vi "PicoScope3000aExampleBlockAdvancedTrig.vi"() -> ()   [LabVIEW 2010]
uses:
  shared/PicoBuffers.ctl
  <vilib>/Waveform/DWDTOps.llb/DWDT Analog to Digital.vi
  shared/Buffer and Transfer Settings.ctl
  shared/Acquisition Settings.ctl
  PicoScope3000aLib/PicoScope3000aDigitalChannelSettings.ctl
  PicoScope3000aLib/PicoScope3000aAnalogChannelSettings.ctl
panel:
  in  "roundFaster":bool=TRUE
  in  "timeIntervalRequested":dbl min=0.0 format="%#6_6p"
  in  "Write to TDMS":bool
  in  "Channel B Trigger Properties":T1={"thresholdUpper"=0, "thresholdUpperHysteresis"=1024, "thresholdLower"=0, "thresholdLowerHysteresis"=1024, "Threshold Mode"=0, "Direction"=2, "Available"=FALSE} {"Direction" items=["Above / Inside", "Below / Outside", "Rising / Enter", "Falling / Exit", "Rising or Falling / Enter or Exit", "Above Lower", "Below Lower", "Rising Lower", "Falling Lower", "Positive Runt", "Negative Runt"]; "Threshold Mode" items=["Level", "Window"]}
  in  "Channel B Settings":T2={"Enabled"=FALSE, "Coupling"=1, "Range"=6, "Analogue Offset"=0.0, "Bandwidth Limit"=0} {"Bandwidth Limit" items=["Full", "20MHz"]; "Range" items=["10 mV", "20 mV", "50 mV", "100 mV", "200 mV", "500 mV", "1 V", "2 V", "5 V", "10 V", "20 V", "50 V ", "100 V"]; "Coupling" items=["AC", "DC"]}
  in  "Pulse Width Qualifier Conditions":T3 {"Condition Logic" items=["AND", "OR", "XOR"]}
  in  "Pulse Width Qualifier Settings":T4={"Direction"=2, "Lower Limit"=0, "Upper Limit"=0, "Pulse Width Type"=0} {"Pulse Width Type" items=["None", "Less Than", "Greater Than", "In Range", "Out of Range"]; "Direction" items=["Rising"=2, "Falling"=3]}
  in  "Auto Trigger (ms)":i32=1000
  in  "Trigger Conditions":T5 {"Condition Logic" items=["AND", "OR", "XOR"]}
  in  "Channel A Trigger Properties":T1={"thresholdUpper"=0, "thresholdUpperHysteresis"=1024, "thresholdLower"=0, "thresholdLowerHysteresis"=1024, "Threshold Mode"=0, "Direction"=2, "Available"=FALSE} {"Direction" items=["Above / Inside", "Below / Outside", "Rising / Enter", "Falling / Exit", "Rising or Falling / Enter or Exit", "Above Lower", "Below Lower", "Rising Lower", "Falling Lower", "Positive Runt", "Negative Runt"]; "Threshold Mode" items=["Level", "Window"]}
  in  "Digital Port  0":T6 {"Direction Channel 7" items=["Don't Care", "Low", "High", "Rising", "Falling"]; "Direction Channel 6" items=["Don't Care", "Low", "High", "Rising", "Falling"]; "Direction Channel 5" items=["Don't Care", "Low", "High", "Rising", "Falling"]; "Direction Channel 4" items=["Don't Care", "Low", "High", "Rising", "Falling"]; "Direction Channel 3" items=["Don't Care", "Low", "High", "Rising", "Falling"]; "Direction Channel 2" items=["Don't Care", "Low", "High", "Rising", "Falling"]; "Direction Channel 1" items=["Don't Care", "Low", "High", "Rising", "Falling"]; "Direction Channel 0" items=["Don't Care", "Low", "High", "Rising", "Falling"]}
  in  "Channel A Settings":T2={"Enabled"=TRUE, "Coupling"=1, "Range"=6, "Analogue Offset"=0.0, "Bandwidth Limit"=0} {"Bandwidth Limit" items=["Full", "20MHz"]; "Range" items=["10 mV", "20 mV", "50 mV", "100 mV", "200 mV", "500 mV", "1 V", "2 V", "5 V", "10 V", "20 V", "50 V ", "100 V"]; "Coupling" items=["AC", "DC"]}
  in  "Port 0 Settings":T7={"Enabled"=FALSE, "Logic Level"=9830} {"Logic Level" items=["1.5V TTL"=9830, "2.5V CMOS"=16383]}
  out "overflow":i16 format="%010b"
  in  "Apply Settings":bool
  out "USB 3.0 device on non-USB 3.0 Port":bool=TRUE
  out "USB Powered":bool=TRUE
  out "Device Info":T8={"Driver Version"="", "USB Version"="", "Hardware"="1", "Variant"="", "Batch and Serial"="", "Cal Date"="", "Kernel Version"="", "Digital HW Version"="", "Analogue HW Version"="", "MSO"=FALSE, "Number of channels"=2}
  out "error out":errorcluster
  in  "Data file":path=path "PicoScope3000aExampleBlock Data"
  in  "Buffer and Transfer Settings":T9={"startIndex"=0, "Samples"=1000000, "Down Sample Ratio"=1, "Down-Sample Mode"=0} {"Down-Sample Mode" items=["RAW none"=2147483648, "None"=0, "Aggregate"=1, "Decimate"=2, "Average"=4]; "Down Sample Ratio" step=1; "Samples" format="%_6p"}
  in  "Acquisition Settings":T10={"preTriggerSamples"=0, "postTriggerSamples"=1000000, "timebase"=0} {"postTriggerSamples" format="%_6p"; "preTriggerSamples" format="%_6p"}
  out "Properties Panel":T11 {"Max Total Capture Time Available (sec)" format="%.3p"; "Sample Frequency" format="%.6p"; "Sample Rate" format="%.3p"; "Max Samples Available" format="%_6p"; "Total Capture Time (sec)" format="%.3p"}
  out "Port 0":digitalwaveform(graph)={"t0"=timestamp(0 s since 1904-01-01), "dt"=8e-09, "Y"={"transitions"=[], "data"=[]}}
  in  "stop":bool
  out "Analog Channels":cluster{i32, sgl, "Data":dbl[]}[](graph)
  in  "Serial Number":string
  in  "Use Serial Number":bool
  in  "error in (no error)":errorcluster
  # "Bit 0 = ChA"
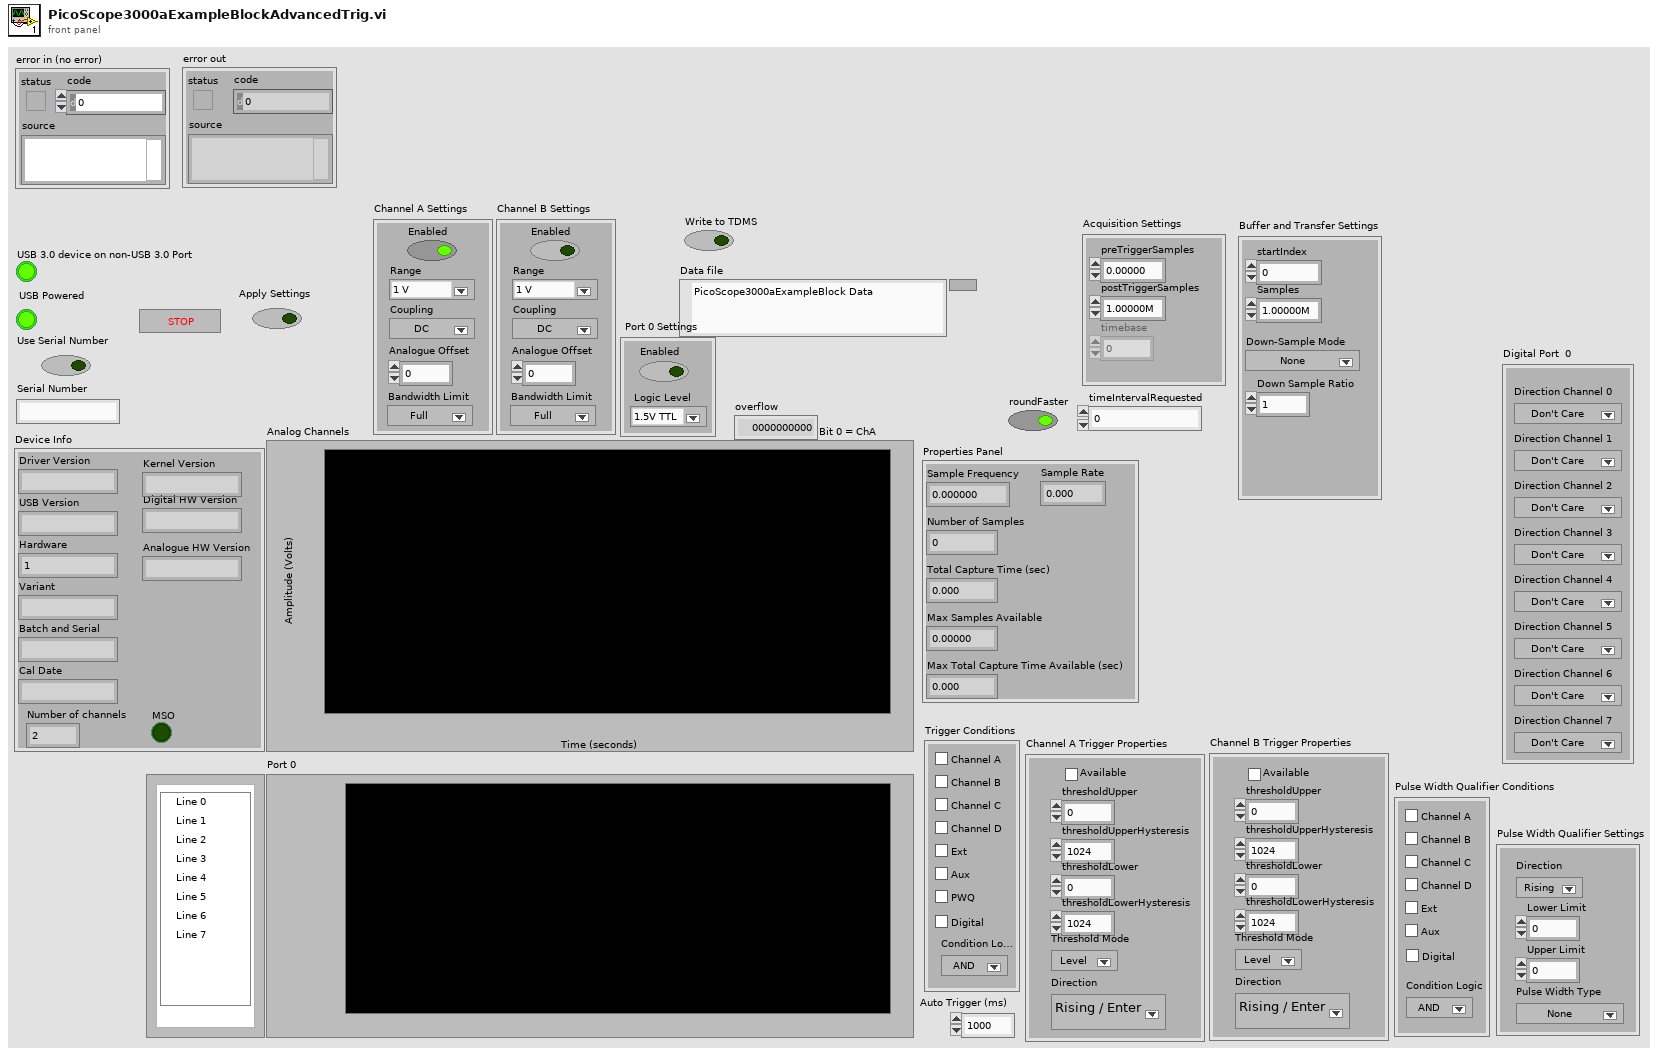
[diagram p1: front panel]
types:
  T1 = cluster{"thresholdUpper":i16, "thresholdUpperHysteresis":u16, "thresholdLower":i16, "thresholdLowerHysteresis":u16, "Threshold Mode":i32, "Direction":i32, "Available":bool}
  T2 = typedef "PicoScope3000aAnalogChannelSettings.ctl" = cluster{"Enabled":bool, "Coupling":u32, "Range":u32, "Analogue Offset":sgl, "Bandwidth Limit":u32}
  T3 = cluster{"Channel A":bool, "Channel B":bool, "Channel C":bool, "Channel D":bool, "Aux":bool, "Condition Logic":u16, "Ext":bool, "Digital":bool}
  T4 = cluster{"Direction":u32, "Lower Limit":u32, "Upper Limit":u32, "Pulse Width Type":u32}
  T5 = cluster{"Channel A":bool, "Channel B":bool, "Channel C":bool, "Channel D":bool, "Aux":bool, "PWQ":bool, "Condition Logic":u16, "Ext":bool, "Digital":bool}
  T6 = cluster{"Direction Channel 0":u16, "Direction Channel 1":u16, "Direction Channel 2":u16, "Direction Channel 3":u16, "Direction Channel 4":u16, "Direction Channel 5":u16, "Direction Channel 6":u16, "Direction Channel 7":u16}
  T7 = typedef "PicoScope3000aDigitalChannelSettings.ctl" = cluster{"Enabled":bool, "Logic Level":i16}
  T8 = cluster{"Driver Version":string, "USB Version":string, "Hardware":string, "Variant":string, "Batch and Serial":string, "Cal Date":string, "Kernel Version":string, "Digital HW Version":string, "Analogue HW Version":string, "MSO":bool, "Number of channels":i16}
  T9 = typedef "Buffer and Transfer Settings.ctl" = cluster{"startIndex":u64, "Samples":u64, "Down Sample Ratio":u64, "Down-Sample Mode":u32}
  T10 = typedef "Acquisition Settings.ctl" = cluster{"preTriggerSamples":u64, "postTriggerSamples":u64, "timebase":u32}
  T11 = cluster{"Sample Frequency":dbl, "Sample Rate":dbl, "Max Samples Available":u64, "Number of Samples":u64, "Total Capture Time (sec) ":dbl, "Max Total Capture Time Available (sec)":dbl}
  T12 = typedef "PicoBuffers.ctl" = cluster{"Max Buffer Pointers":u64[][][], "Min Buffer Pointers":u64[][][], "StreamingDataInfo":cluster{"Channel":u32, "Down-Sample Mode":u32, "PICO_DATA_TYPE":enum32{"PICO_INT8_T", "PICO_INT16_T", "PICO_INT32_T", "PICO_UINT32_T", "PICO_INT64_T", ""}, "Samples":i32, "bufferIndex":u64, "startIndex":i32, "overflow":i16}[][]}
  T13 = enum16{"open", "open or create", "create or replace", "create", "open (read-only)"}
  T14 = cluster{"Sample Frequency":sgl, "Sample Rate":sgl, "Max Samples Available":i32, "Number of Samples":u32, "Total Capture Time (sec) ":sgl, "Max Total Capture Time Available (sec)":sgl}
  T15 = cluster{"Channel A Buffer":i16[], "Channel B Buffer":i16[], "Channel C Buffer":i16[], "Channel D Buffer":i16[], "Channel E Buffer":i16[], "Channel F Buffer":i16[], "Channel G Buffer":i16[], "Channel H Buffer":i16[], "Port 0 Buffer":i16[], "Port 1 Buffer":i16[]}[]
  T16 = cluster{"Channel A Buffer":i16[], "Channel B Buffer":i16[], "Channel C Buffer":i16[], "Channel D Buffer":i16[], "Channel E Buffer":i16[], "Channel F Buffer":i16[], "Channel G Buffer":i16[], "Channel H Buffer":i16[], "Port 0 Buffer":i16[], "Port 1 Buffer":i16[]}
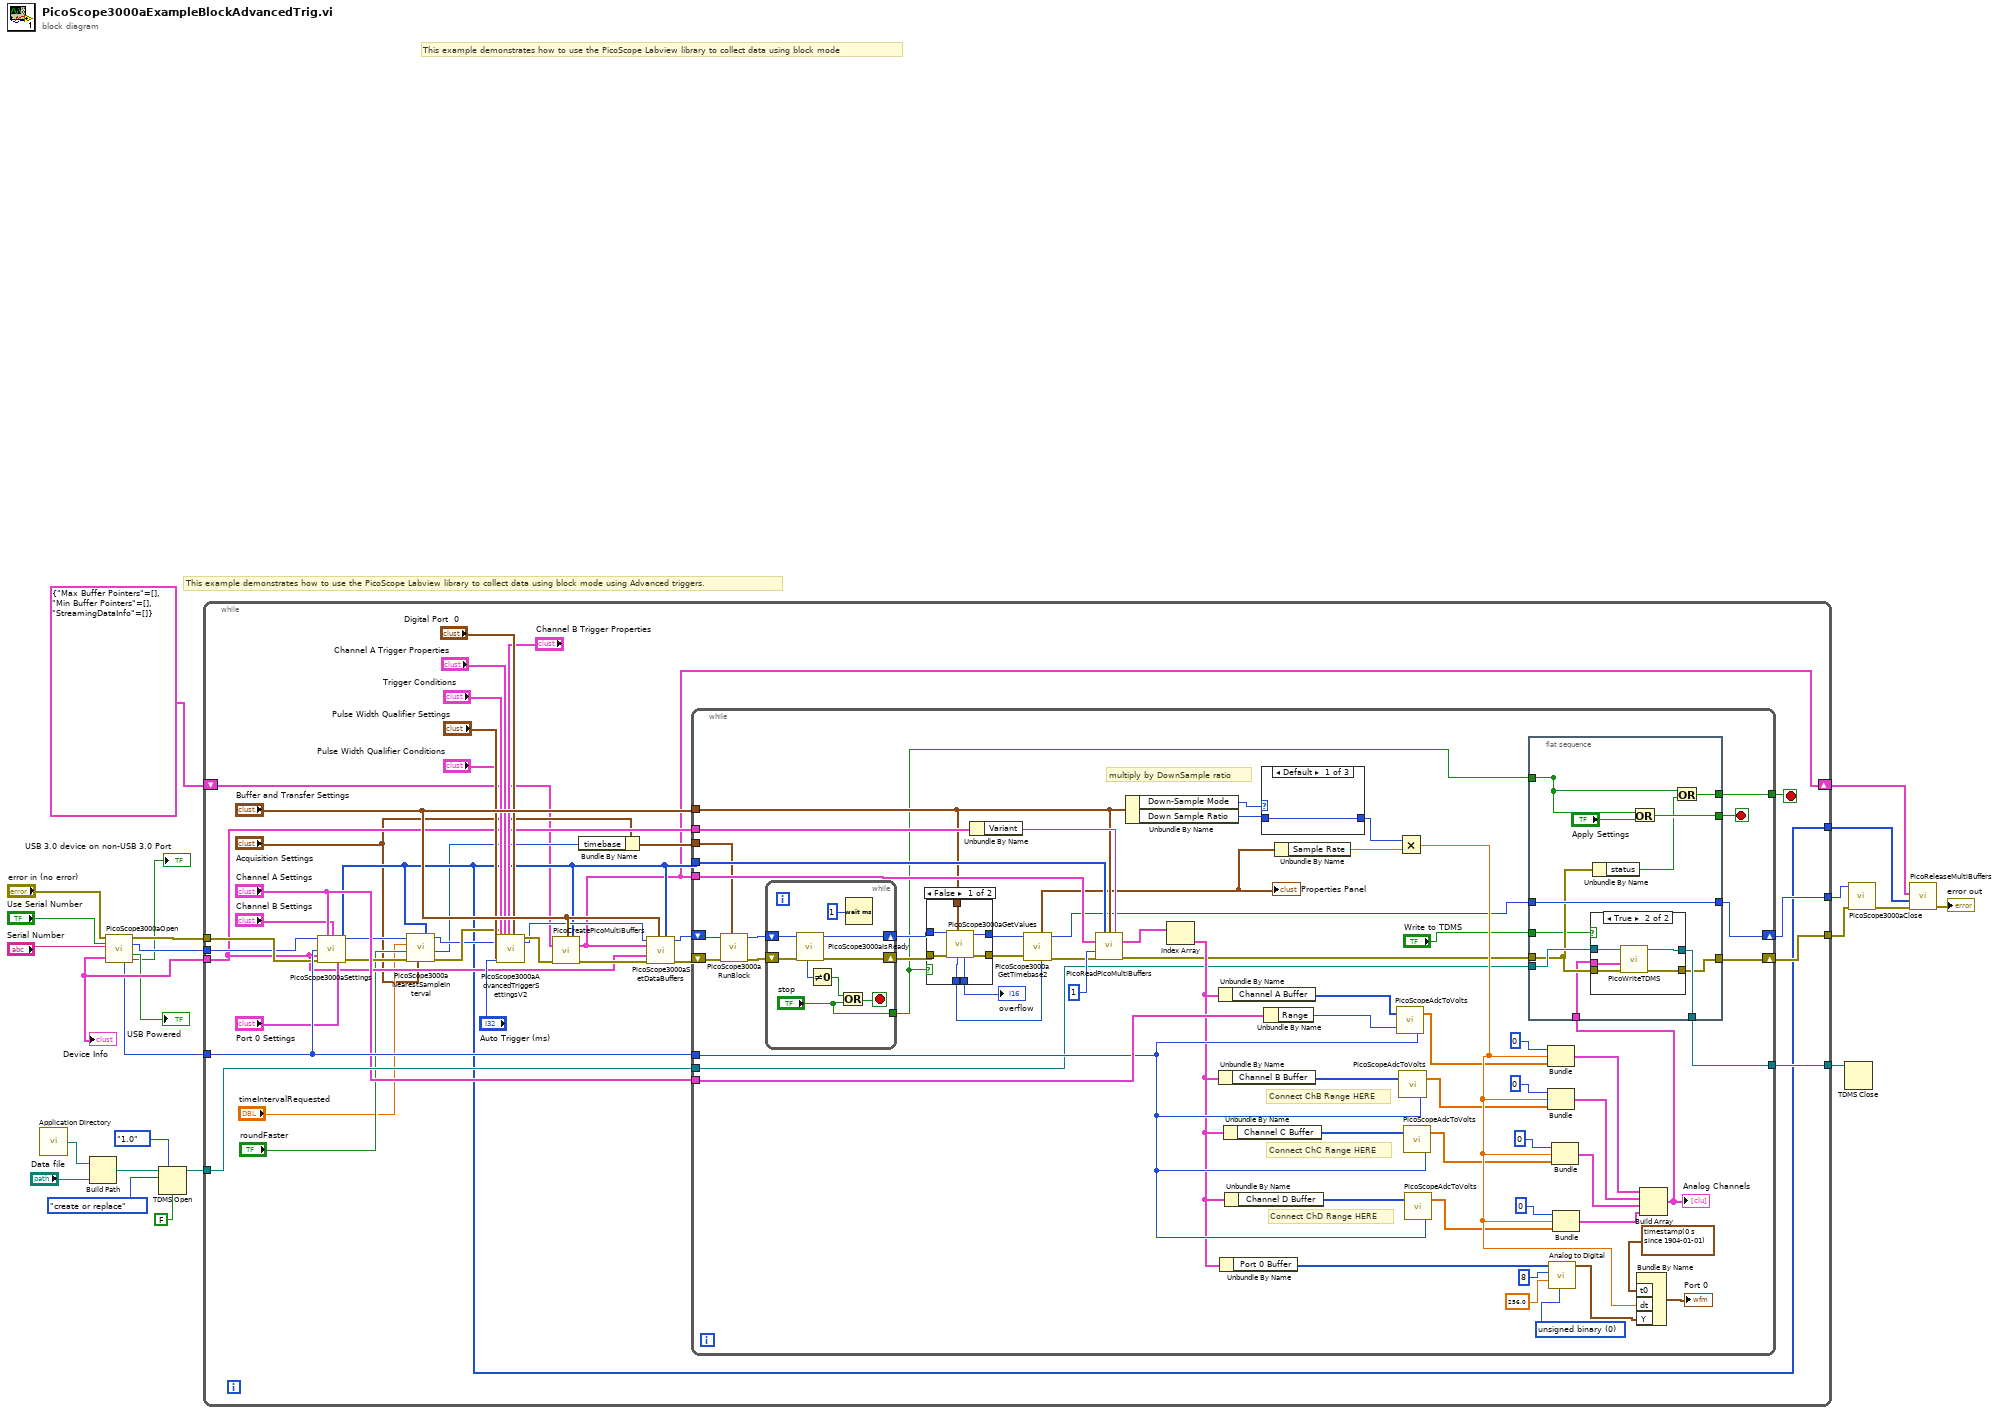
[diagram p0: block diagram]
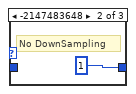
[diagram p4: hidden frame]
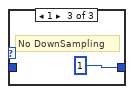
[diagram p5: hidden frame]
diagram:
  # "This example demonstrates how to use the PicoScope Labview library to collect data using block mode using Advanced triggers."
  # "This example demonstrates how to use the PicoScope Labview library to collect data using block mode"
  n1 = call <vilib>:"Application Directory.vi"() -> ("Application Directory"=w17:path)
  n2 = Build Path(base path=w17, name or relative path="Data file") -> (appended path=w18:path)
  n3 = call "PicoScope3000aOpen.vi"("error in (no error)"="error in (no error)", "Serial Number"="Serial Number", "Use Serial number"="Use Serial Number") -> ("error out"=w8:errorcluster, "handle"=w24:i16, "USB Powered"=→"USB Powered":bool, "Device Info"=w10:T8, "Max ADC value"=w6:i16, "USB 3.0 device on non-USB 3.0 Port"=→"USB 3.0 device on non-USB 3.0 Port":bool)  [unwired: 6 in, 1 out]
  "Device Info" <- w10
  n4 = TDMS Open(6:FALSE ("disable buffering? (T)"), 7:enum16{"1.0", "2.0"}."1.0" ("file format version (2.0)"), 10:T13."create or replace" ("operation (0:open)"), 11:w18) -> (3:w15:refnum<k34>)  [unwired: 2 in, 1 out]
  n5 = while {
    tunnel: w24 -> [w40]
    tunnel: w6 -> [w52]
    tunnel: [w30] -> w23
    tunnel: [w58] -> w16
    tunnel: w15 -> [w60]
    tunnel: w10 -> [w37]
    tunnel: w8 -> [w41]
    tunnel: [w59] -> w4
    tunnel: [w56] -> w7
    shift-right: [w25] -> w1
    shift-left: T12 {"Max Buffer Pointers"=[], "Min Buffer Pointers"=[], "StreamingDataInfo"=[]} ("Data Pointers") -> [w26]
    stop <- w57 stop-if-true
    n6 = call "PicoScope3000aSettings.vi"("handle in"=w40, "Channel A Settings"="Channel A Settings", "Channel B Settings"="Channel B Settings", "Port 0 Settings"="Port 0 Settings", "Max_adc"=w52, "Device Info"=w37, "error in"=w41) -> ("handle out"=w34:i16, "Enabled Array"=w30:i16[], "error out"=w36:errorcluster)  [unwired: 6 in]
    n7 = call "PicoScope3000aNearestSampleInterval.vi"("Enabled array"=w30, "Acquisition Settings"="Acquisition Settings", "error in (no error)"=w36, "roundFaster"="roundFaster", "timeIntervalRequested"="timeIntervalRequested", "handle in"=w34) -> ("error out"=w32:errorcluster, "timebase"=w27:u32, "handle out"=w31:i16)  [unwired: 2 in, 1 out]
    n8 = call "PicoScope3000aAdvancedTriggerSettingsV2.vi"("error in"=w32, "handle in"=w31, "Trigger Conditions"="Trigger Conditions", "Auto Trigger (ms)"="Auto Trigger (ms)", "Channel A Trigger Properties"="Channel A Trigger Properties", "Channel B Trigger Properties"="Channel B Trigger Properties", "Digital Port  0"="Digital Port  0", "Pulse Width Qualifier Conditions"="Pulse Width Qualifier Conditions", "Pulse Width Qualifier Settings"="Pulse Width Qualifier Settings") -> ("error out"=w49:errorcluster, "handle out"=w48:i16)  [unwired: 9 in]
    n9 = call "PicoCreatePicoMultiBuffers.vi"("Buffer and Transfer Settings"="Buffer and Transfer Settings", "enabled array"=w30, "Data Pointers In"=w26, "error in (no error)"=w49) -> ("Data Pointers"=w25:T12, "error out"=w61:errorcluster)  [unwired: 10 in]
    n10 = Bundle By Name(cluster="Acquisition Settings", "timebase"=w27) -> (w29:T10)
    n11 = call "PicoScope3000aSetDataBuffers.vi"("enabled array"=w30, "Buffer and Transfer Settings"="Buffer and Transfer Settings", "error in (no error)"=w61, "Device Info"=w37, "Data Pointers In"=w25, "handle in"=w48) -> ("error out"=w55:errorcluster, "handle out"=w54:i16)  [unwired: 4 in]
    n12 = while {
      tunnel: w25 -> [w124]
      tunnel: "Buffer and Transfer Settings" -> [w74]
      tunnel: w30 -> [w116]
      tunnel: "Channel A Settings" -> [w115]
      tunnel: w29 -> [w114]
      tunnel: w52 -> [w113]
      tunnel: w37 -> [w110]
      tunnel: [w81] -> w57
      shift-right: [w83] -> w59
      shift-left: w55 -> [w75]
      shift-right: [w79] -> w56
      shift-left: w54 -> [w76]
      tunnel: w60 -> [w65]
      tunnel: [w64] -> w58
      stop <- w80 stop-if-true
      w100 = u16 0 items=["unsigned binary", "offset binary", "2's complement"] ("data format (offset binary)")
      # "Connect ChB Range HERE"
      # "Connect ChD Range HERE"
      # "Connect ChC Range HERE"
      # "multiply by DownSample ratio"
      n13 = call "PicoScope3000aRunBlock.vi"("Acquisition Settings"=w114, "error in (no error)"=w75, "handle in"=w76) -> ("error out"=w118:errorcluster, "handle out"=w117:i16)  [unwired: 5 in, 2 out]
      n14 = while {
        shift-right: [w160] -> w77
        shift-left: w118 -> [w161]
        shift-right: [w159] -> w78
        shift-left: w117 -> [w158]
        tunnel: ["stop"] -> w73
        stop <- w155 stop-if-true
        n15 = call "PicoScope3000aIsReady.vi"("error in (no error)"=w161, "handle in"=w158) -> ("error out"=w160:errorcluster, "handle out"=w159:i16, "ready"=w157:i16)  [unwired: 7 in]
        n16 = Not Equal To 0?(x=w157) -> (x != 0?=w156:bool)
        n17 = Or(x=w156, y="stop") -> (x .or. y?=w155:bool)
        n18 = Wait (ms)(milliseconds to wait=u32 1) -> ()  [unwired: 1 out]
      }
      n19 = case shown="False" w73 {
        tunnel: w77 -> [w131 w132]
        tunnel: w78 -> [w130 w133]
        tunnel: [w129 w133] -> w68
        tunnel: [w128 w132] -> w69
        tunnel: w74 -> [w127 _]
        tunnel: [w126 _] -> w72
        tunnel: [w125 _] -> w71
        frame False {
          n20 = call "PicoScope3000aGetValues.vi"("Buffer and Transfer Settings"=w127, "error in (no error)"=w131, "handle in"=w130) -> ("error out"=w128:errorcluster, "handle out"=w129:i16, "overflow"=w126:i16, "noOfSamples"=w125:u64)  [unwired: 5 in]
        }
        frame True {
        }
      }
      "overflow" <- w72
      n21 = Unbundle By Name(w110) -> ("Variant"=w111:string)
      n22 = call "PicoScope3000aGetTimebase2.vi"("Number of Samples"=w71, "error in (no error)"=w69, "handle in"=w68) -> ("error out"=w67:errorcluster, "handle out"=w66:i16, "Properties Panel"=w70:T14)  [unwired: 6 in]
      "Properties Panel" <- w70
      n23 = call "PicoReadPicoMultiBuffers.vi"("enabled array"=w116, "Buffer and Transfer Settings"=w74, "Variant"=w111, "Data Pointers"=w124, "No of Buffers"=1, "error in (no error)"=w67) -> ("MultiBuffers (Max or non-aggregated)"=w123:T15, "error out"=w82:errorcluster)  [unwired: 7 in, 1 out]
      n24 = Unbundle By Name(w74) -> ("Down-Sample Mode"=w121:u32, "Down Sample Ratio"=w122:u64)
      n25 = Index Array(array=w123) -> (element=w84:T16)  [unwired: 1 in]
      n26 = Unbundle By Name(w84) -> ("Channel A Buffer"=w93:i16[])
      n27 = Unbundle By Name(w84) -> ("Channel B Buffer"=w105:i16[])
      n28 = Unbundle By Name(w84) -> ("Port 0 Buffer"=w98:i16[])
      n29 = Unbundle By Name(w84) -> ("Channel C Buffer"=w91:i16[])
      n30 = Unbundle By Name(w84) -> ("Channel D Buffer"=w87:i16[])
      n31 = case shown="Default" w121 {
        tunnel: [w162 u64 1 ("Down Sample Ratio") u64 1 ("Down Sample Ratio")] -> w119
        tunnel: w122 -> [w162 _ _]
        frame Default {
        }
        frame -2147483648 {
          # "No DownSampling"
        }
        frame 1 {
          # "No DownSampling"
        }
      }
      n32 = Unbundle By Name(w115) -> ("Range"=w107:u32)
      n33 = Unbundle By Name(w70) -> ("Sample Rate"=w112:sgl)
      n34 = call "PicoScopeAdcToVolts.vi"("Max_adc"=w113, "Range Index"=w107, "Data"=w93) -> ("Data"=w94:dbl[])
      n35 = Multiply(x=w119, y=w112) -> (x*y=w120:sgl)
      n36 = call "PicoScopeAdcToVolts.vi"("Max_adc"=w113, "Data"=w105) -> ("Data"=w104:dbl[])  [unwired: 1 in]
      n37 = call "PicoScopeAdcToVolts.vi"("Max_adc"=w113, "Data"=w91) -> ("Data"=w90:dbl[])  [unwired: 1 in]
      n38 = call "PicoScopeAdcToVolts.vi"("Max_adc"=w113, "Data"=w87) -> ("Data"=w86:dbl[])  [unwired: 1 in]
      n39 = flat-sequence {
        tunnel: [w145] -> w80
        tunnel: [w140] -> _
        tunnel: [w142] -> w81
        tunnel: w66 -> [w141]
        tunnel: [w141] -> w79
        tunnel: w82 -> [w136]
        tunnel: [w137] -> w83
        tunnel: w73 -> [w140]
        tunnel: w65 -> [w139]
        tunnel: [w138] -> w64
        tunnel: w63 -> [w135]
        tunnel: "Write to TDMS" -> [w134]
        frame #0 {
          n40 = case shown="True" w134 {
            tunnel: w135 -> [_ w152]
            tunnel: w139 -> [w146 w151]
            tunnel: w136 -> [w147 w150]
            tunnel: [w147 w149] -> w137
            tunnel: [w146 w148] -> w138
            frame False {
            }
            frame True {
              n41 = call "PicoWriteTDMS.vi"("error in (no error)"=w150, "Analog Channels"=w152, "Refnum in"=w151) -> ("error out"=w149:errorcluster, "Refnum out"=w148:refnum<k34>)  [unwired: 7 in]
            }
          }
          n42 = Unbundle By Name(w136) -> ("status"=w143:bool)
          n43 = Or(x=w140, y="Apply Settings") -> (x .or. y?=w145:bool)
          n44 = Or(x=w140, y=w143) -> (x .or. y?=w142:bool)
        }
      }
      n45 = Bundle(0, w120, "Data"=w94) -> (w103:cluster{i32, sgl, "Data":dbl[]})  [unwired: 1 in]
      n46 = Bundle(0, w120, "Data"=w104) -> (w102:cluster{i32, sgl, "Data":dbl[]})  [unwired: 1 in]
      n47 = call-poly <vilib>:"Analog to Digital.vi"("data format (offset binary)"=w100, "full-scale range (pk-pk)"=256.0, "resolution (16 bit)"=8, "analog waveform"=w98) -> ("digital waveform"=w95:digitalwaveform)  [unwired: 4 in, 3 out]
      n48 = Bundle(0, w120, "Data"=w90) -> (w89:cluster{i32, sgl, "Data":dbl[]})  [unwired: 1 in]
      n49 = Bundle(0, w120, "Data"=w86) -> (w85:cluster{i32, sgl, "Data":dbl[]})  [unwired: 1 in]
      n50 = Bundle By Name("t0"=timestamp(0 s since 1904-01-01), "dt"=w120, "Y"=w95) -> (→"Port 0":digitalwaveform)  [unwired: 1 in]
      n51 = Build Array(w103, w102, w89, w85) -> (w63:cluster{i32, sgl, "Data":dbl[]}[])
      "Analog Channels" <- w63
    }
  }
  n52 = TDMS Close(11:w16) -> ()  [unwired: 1 in, 2 out]
  n53 = call "PicoScope3000aClose.vi"("error in (no error)"=w4, "handle in"=w7) -> ("error out"=w3:errorcluster)  [unwired: 8 in, 1 out]
  n54 = call "PicoReleaseMultiBuffers.vi"("error in (no error)"=w3, "Enabled array"=w23, "Data Pointers"=w1) -> ("error out"=→"error out":errorcluster)  [unwired: 7 in, 1 out]
